vi "RVC Roll-Pitch-Yaw Transformation.vi"() -> ()   [LabVIEW 2013]
uses:
  <vilib>/robotics/Kinematics/NI_Kinematics.lvlib
panel:
  in  "Convension":u16(ring) items=["XYZ", "ZYX"]
  out "gamma (euler angles)":T1
  out "transformation matrix":picture
  in  "Position":dbl[](array[numeric])=[1.0, 1.0, 1.0]
  in  "angles":cluster{"roll":dbl, "pitch":dbl, "yaw":dbl}={"roll"=0.1, "pitch"=0.2, "yaw"=0.3} {"roll" scale=-3.14..3.14; "pitch" scale=-1.54..1.54; "yaw" scale=-3.14..3.14}
  out "3D Picture":refnum<vi>(3d-picture)
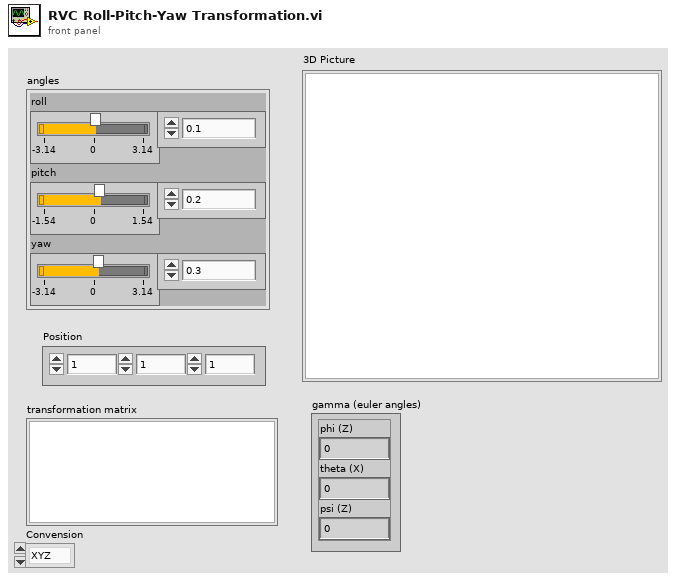
[diagram p1: front panel]
types:
  T1 = cluster{"phi (Z)":dbl, "theta (X)":dbl, "psi (Z)":dbl}
  T2 = typedef "NI_Matrix.lvlib/RealMatrix.ctl" = dbl[][]
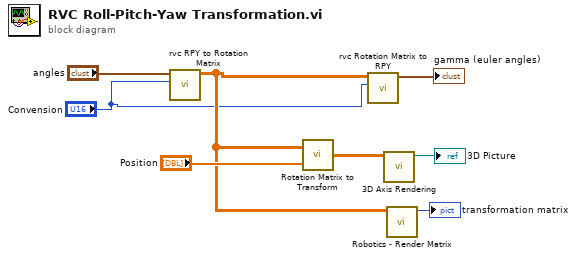
[diagram p0: block diagram]
diagram:
  n1 = call "rvc RPY to Rotation Matrix.vi"("Convension"="Convension", "angles"="angles") -> ("rotation matrix"=w2:T2)  [unwired: 9 in]
  n2 = call <vilib>:"Rotation Matrix to Transform.vi"("translation vector"="Position", "rotation matrix"=w2) -> ("transform"=w7:T2)
  n3 = call "rvc Rotation Matrix to RPY.vi"("Convension"="Convension", "rotation matrix"=w2) -> ("angles"=→"gamma (euler angles)":cluster{"roll":dbl, "pitch":dbl, "yaw":dbl})  [unwired: 9 in]
  n4 = call "3D Axis Rendering.vi"("rotation matrix"=w7) -> ("SceneNode out"=→"3D Picture":refnum<vi>)  [unwired: 9 in, 1 out]
  n5 = call "Robotics - Render Matrix.vi"("A"=w2) -> ("picture out"=→"transformation matrix":picture)  [unwired: 10 in]
